vi "Fix Variable Name.vi"(11 "Variable in":string) -> (3 "Variable out":string)   [LabVIEW 2020, in "Output Sequencer.lvlib" / "Output Sequencer.lvclass"]
uses:
  Output Sequencer.lvclass
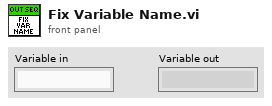
[diagram p1: front panel]
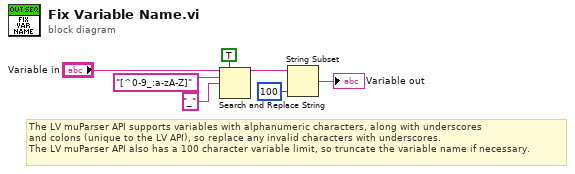
[diagram p0: block diagram]
diagram:
  # "The LV muParser API supports variables with alphanumeric characters, along with underscores\nand colons (unique to the LV API), so replace any invalid characters with underscores.\nThe LV muParser API also has a 100 character variable limit, so truncate the variable name if necessary."
  n1 = Search and Replace String(replace all?=TRUE ("replace all? (F)"), input string="Variable in", search string="[^0-9_:a-zA-Z]" ("Regex"), replace string="_" ("replace string (\"\")")) -> (result string=w5:string)  [unwired: 4 in, 3 out]
  n2 = String Subset(string=w5, length (rest)=100 ("length (rest)")) -> (substring=→"Variable out":string)  [unwired: 1 in]
